vi "Kill LV.vi"(8 "error in (no error)":errorcluster) -> (0 "error out":errorcluster, 3 "Output":string)   [LabVIEW 2024, in "Wordle Scorer.lvlib"]
uses:
  Wordle Scorer.lvlib
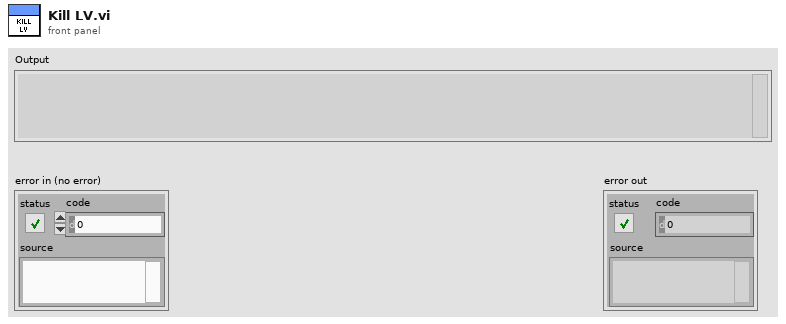
[diagram p1: front panel]
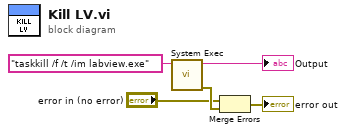
[diagram p0: block diagram]
diagram:
  n1 = call <vilib>:"System Exec.vi"("command line"="taskkill /f /t /im labview.exe") -> ("error out"=w3:errorcluster, "standard output"=→"Output":string)  [unwired: 7 in, 2 out]
  n2 = Merge Errors("error in (no error)", w3) -> (→"error out":errorcluster)
